vi "UMLEditor EscapeHTTPParam.vi"(1 "string":string) -> (0 "url-encoded string":string)   [LabVIEW 2014]
doc: "URL-encodes characters according to RFC 1738.\n\nAll characters, except for alphanumerics and underscore, are replaced with %xx, where xx is the character's hexadecimal value."
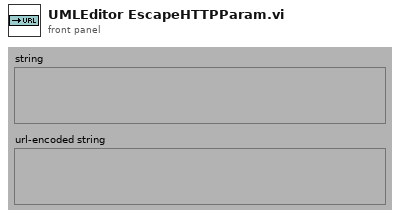
[diagram p1: front panel]
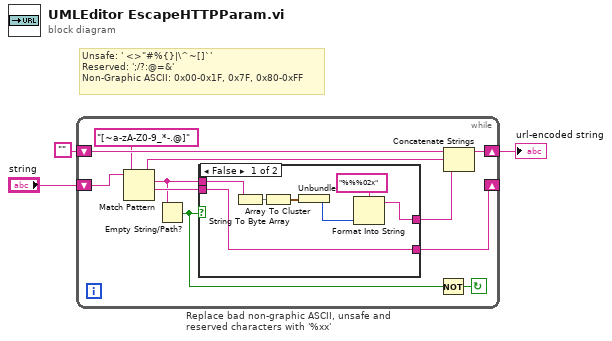
[diagram p0: block diagram]
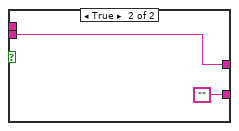
[diagram p2: hidden frame]
diagram:
  # "Unsafe: ' <>\"#%{}|\\^~[]`'\nReserved: ';/?:@=&'\nNon-Graphic ASCII: 0x00-0x1F, 0x7F, 0x80-0xFF"
  n1 = while "Replace bad non-graphic ASCII, unsafe and reserved characters with '%xx'" {
    shift-left: "" -> [w13]
    shift-right: [w11] -> w2
    shift-left: "string" -> [w14]
    shift-right: [w7] -> _
    stop <- w10 continue-if-true
    n2 = Match Pattern(string=w14, regular expression="[~a-zA-Z0-9_*-.@]") -> (before substring=w12:string, match substring=w5:string, after substring=w8:string)  [unwired: 2 out]
    n3 = Empty String/Path?(string/path=w5) -> (empty?=w9:bool)
    n4 = case shown="False" w9 {
      tunnel: w8 -> [w15 w23]
      tunnel: [w15 ""] -> w7
      tunnel: [w20 w23] -> w6
      tunnel: w5 -> [w19 _]
      frame False {
        n5 = String To Byte Array(string=w19) -> (unsigned byte array=w18:u8[])
        n6 = Array To Cluster(array=w18) -> (cluster=w17:cluster{"unsigned byte array[0]":u8})
        n7 = Unbundle(w17) -> ("unsigned byte array[0]"=w16:u8)
        n8 = Format Into String(format string="%%%02x", w16) -> (resulting string=w20:string)  [unwired: 2 in, 1 out]
      }
      frame True {
      }
    }
    n9 = Not(x=w9) -> (.not. x?=w10:bool)
    n10 = Concatenate Strings(w13, w12, w6) -> (w11:string)
  }
  "url-encoded string" <- w2
